vi "dialisis.vi"() -> ()   [LabVIEW 2014]
panel:
  out "T1":bool
  out "T2":bool
  out "TOXINS":dbl
  out "TOXINS":dbl(slide) scale=0.0..2000.0
  out "MILILITERS WATER":dbl
  out ".":bool
  out "1":bool
  out "Water to\nDialyzer":dbl(slide) scale=0.0..6000.0
  out "Boolean 4":bool
  out "Boolean 3":bool
  out "Boolean 2":bool
  out "Boolean":bool
  out "Manometer\nVenous Pressure\nmmHg":dbl(knob) scale=0.0..330.0
  out "Alarm V.P":bool
  in  "Venous\nPressure\nmmHg":dbl
  out "Alarm A.P":bool
  in  "Arterial\nPressure\nmmHg":dbl
  out "Manometer\nArterial Pressure\nmmHg":dbl(knob) scale=0.0..330.0
  out "TOXINES":dynamicdata(graph)
  out "MILILITERS\n VENOUS \nBLOOD":dbl
  out "MILILITERS\nARTERIAL\nBLOOD":dbl
  out "RETURN BLOOD WITH OUT TOXINS":dynamicdata(graph)
  out "FLOW BLOOD WITH TOXINS":dynamicdata(graph)
  in  "ON":bool
  out "Alarm TEMP":bool
  out "Thermometer":dbl(slide) scale=0.0..42.0
  out "Valve return blood":bool
  in  "BLOOD RETURN":dbl
  out "Air Valve":bool
  in  "Air Detector":bool
  out "MOTOR":bool
  in  "OFF":bool
  in  "INITIAL VALUE\nBLOD \nPATIENT":dbl
  out "Venous Blood":dbl(slide) scale=0.0..6000.0
  out "Arterial Blood":dbl(slide) scale=0.0..6000.0
  out "Valve":bool
  # "HEMODIALISIS MACHINE"
  # "HEMODIALYSIS\n MACHINE"
  # "Peristaltic motor"
  # "DIALYZER"
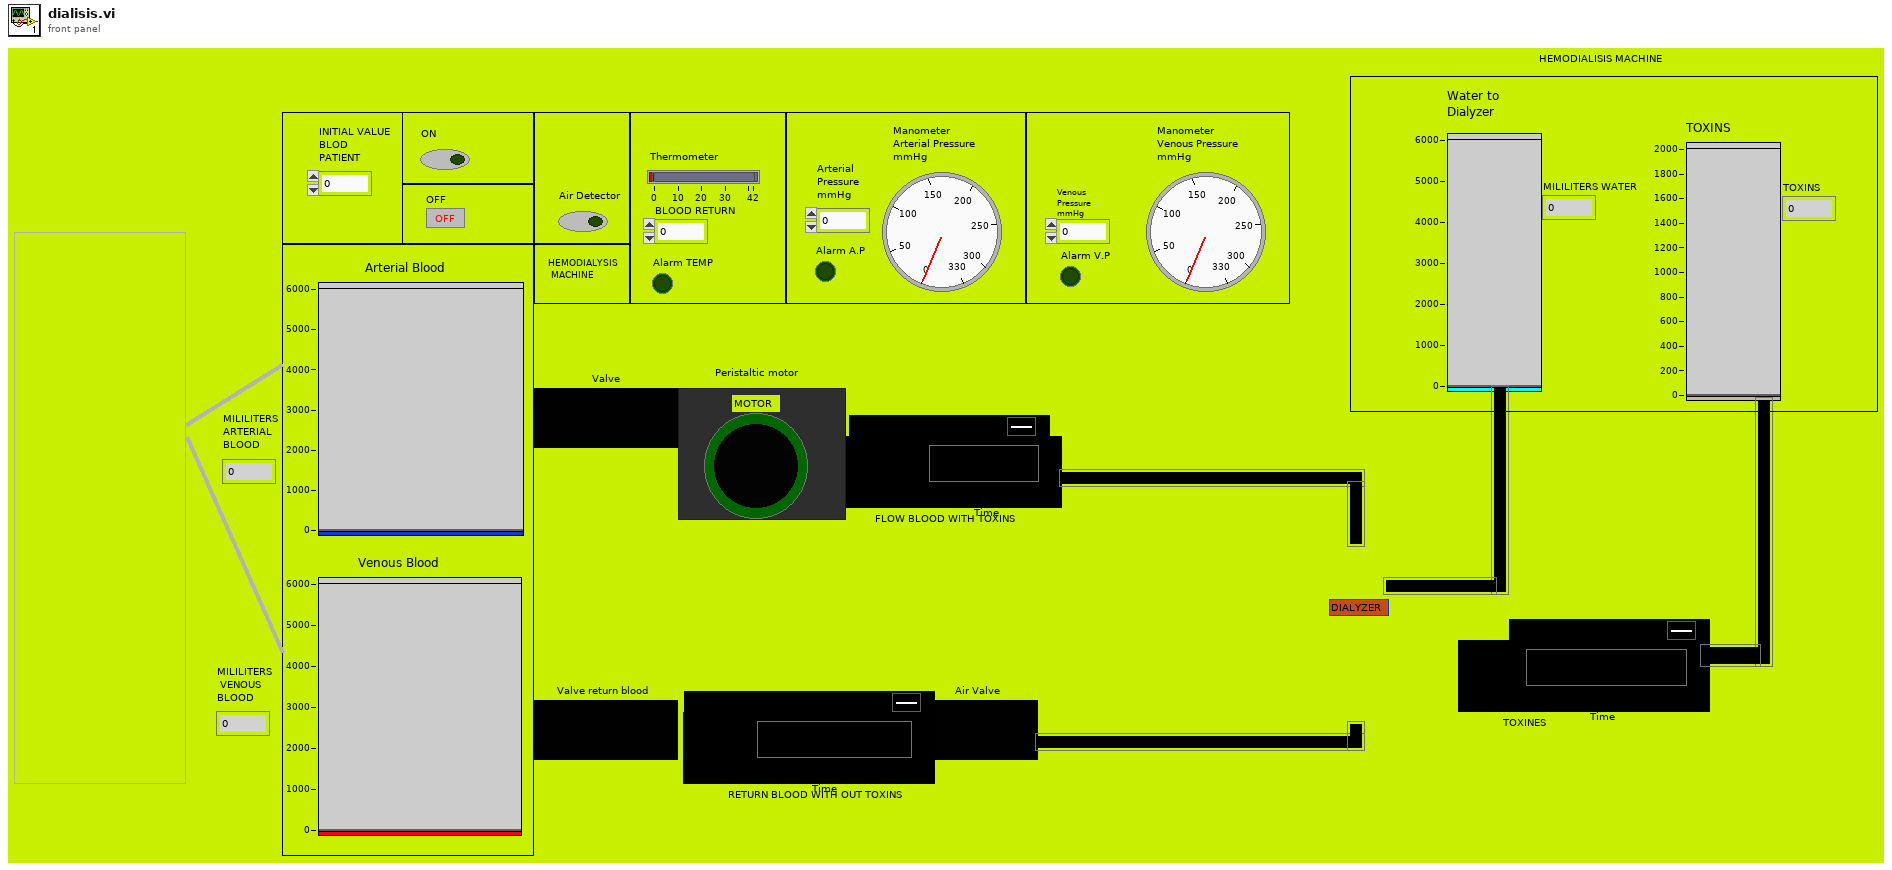
[diagram p1: front panel]
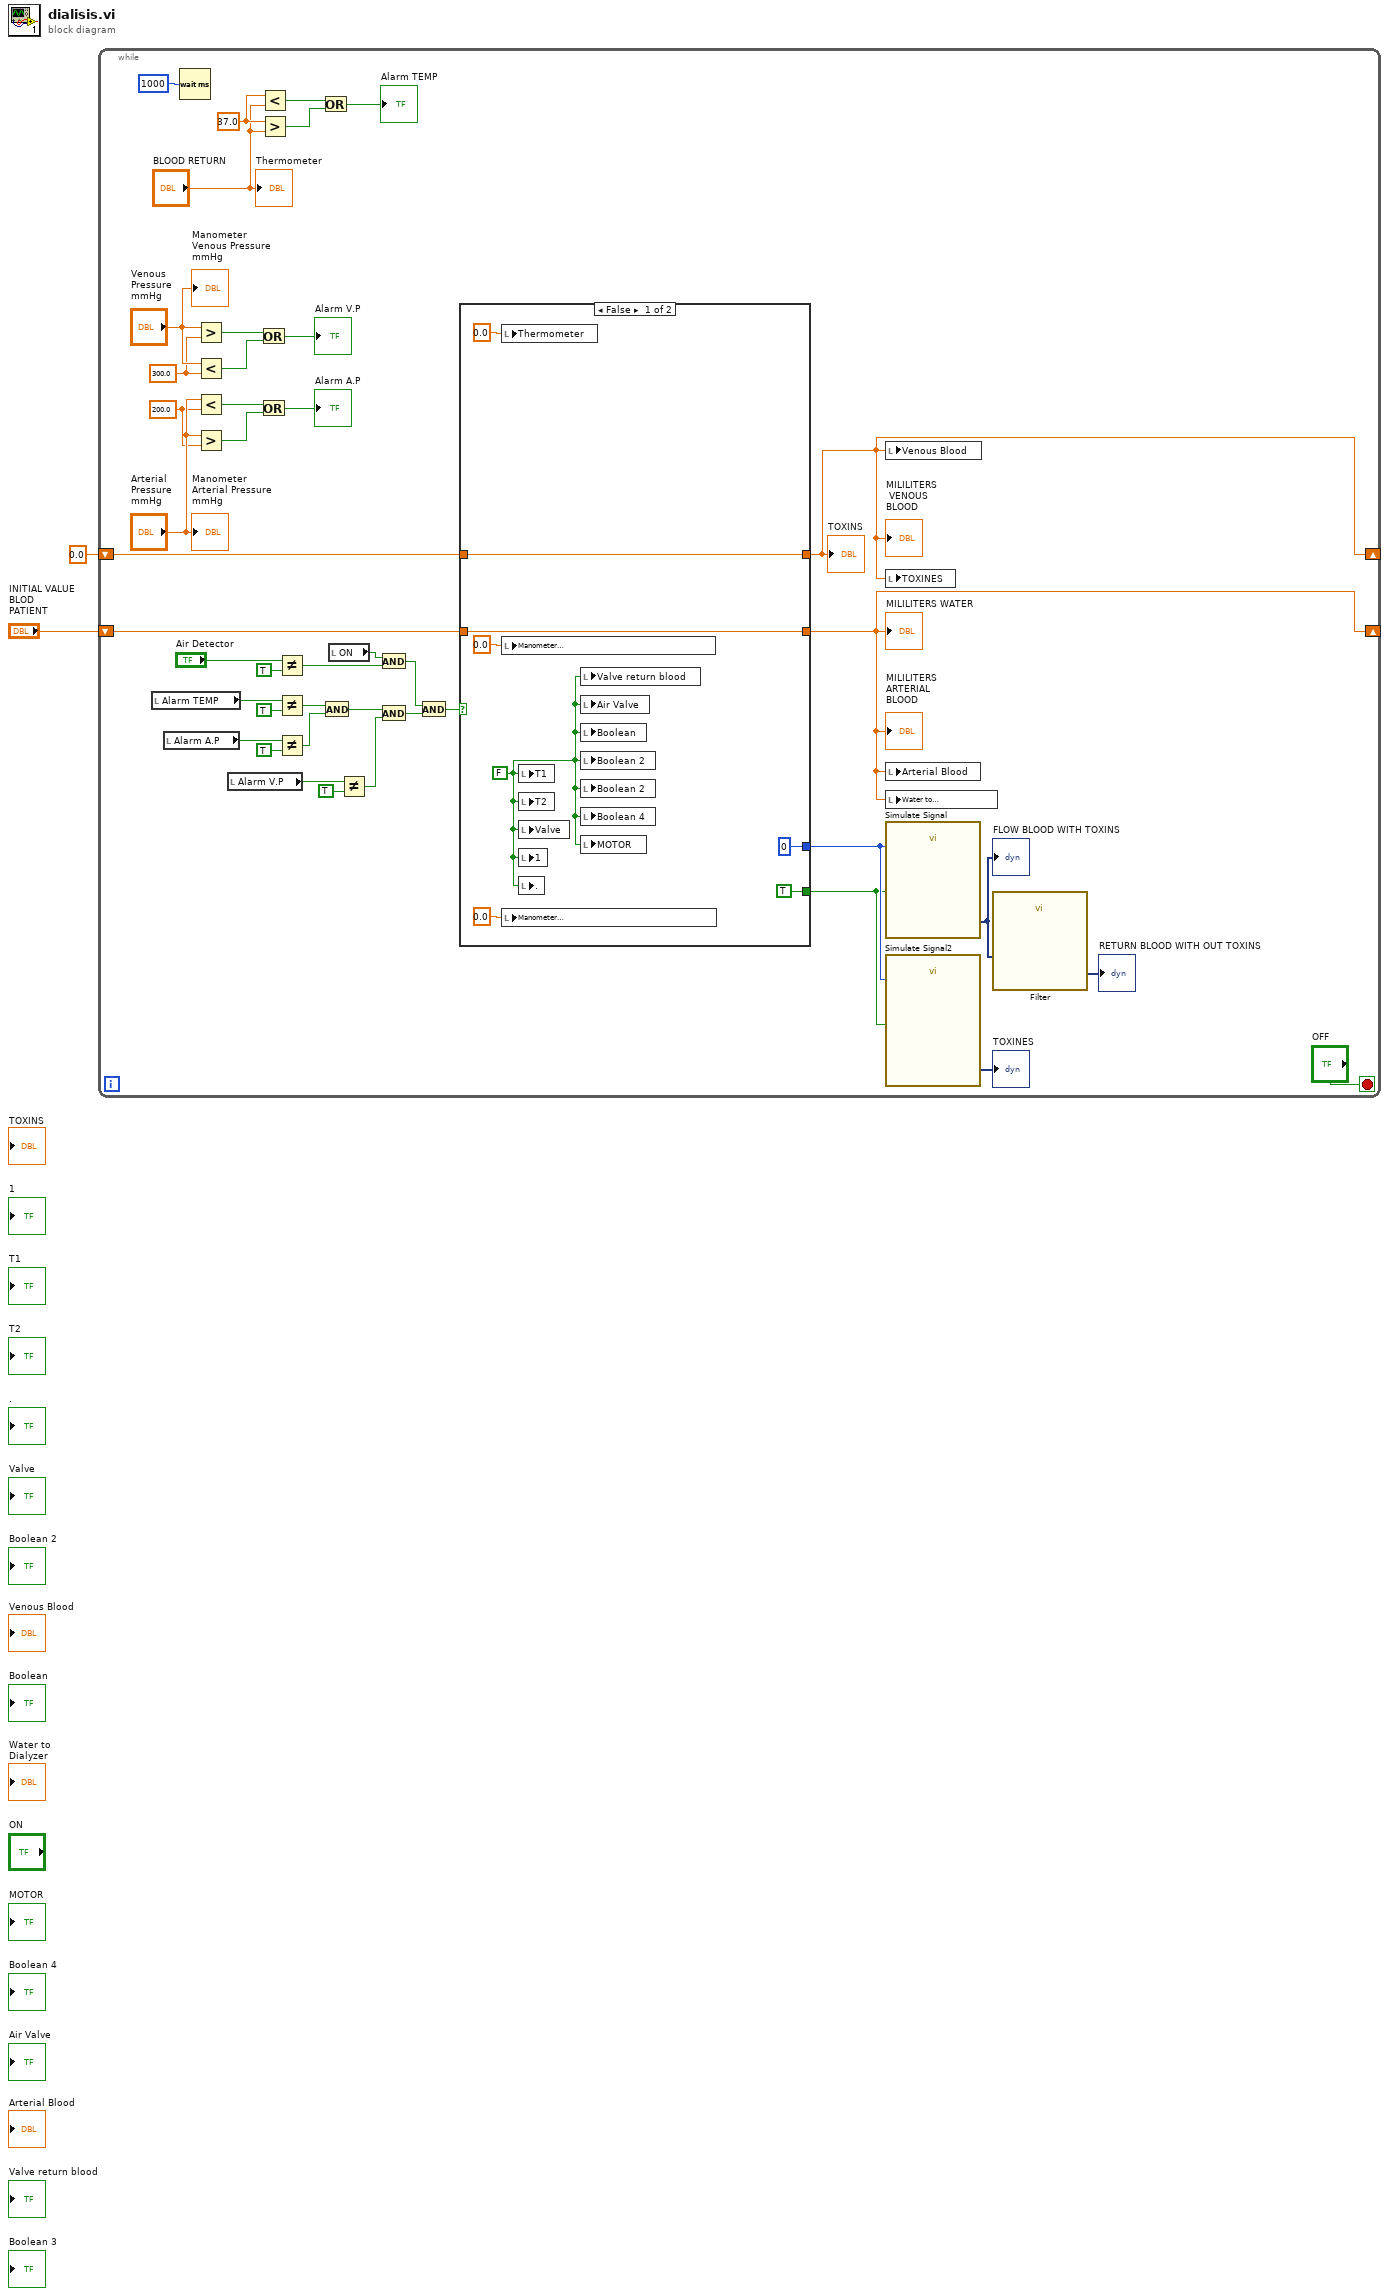
[diagram p0: block diagram]
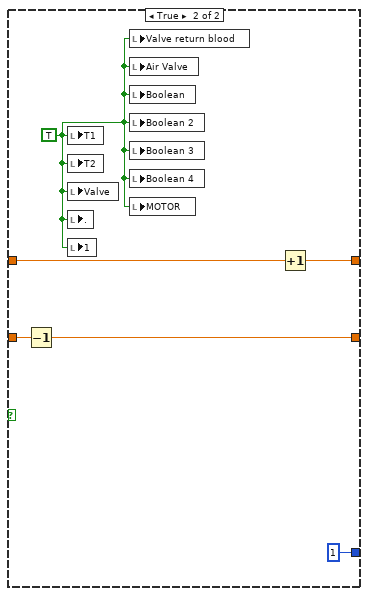
[diagram p2: hidden frame]
diagram:
  n1 = while {
    shift-right: [w5] -> _
    shift-left: "INITIAL VALUE\nBLOD \nPATIENT" -> [w37]
    shift-right: [w3] -> _
    shift-left: 0.0 -> [w4]
    stop <- "OFF" stop-if-true
    w20 = 300.0 ("y")
    w13 = 200.0 ("y")
    w32 = 37.0 ("x")
    n2 = local read "Alarm TEMP"() -> (w35:bool)
    n3 = local read "Alarm A.P"() -> (w25:bool)
    n4 = Wait (ms)(milliseconds to wait=u32 1000) -> ()  [unwired: 1 out]
    n5 = Greater?(x="Venous\nPressure\nmmHg", y=w20) -> (0:w12:bool)
    n6 = Less?(x="Venous\nPressure\nmmHg", y=w20) -> (x < y?=w11:bool)
    n7 = Less?(x="Arterial\nPressure\nmmHg", y=w13) -> (x < y?=w9:bool)
    n8 = Greater?(x="Arterial\nPressure\nmmHg", y=w13) -> (0:w8:bool)
    n9 = local read "Alarm V.P"() -> (w19:bool)
    n10 = Or(x=w12, y=w11) -> (x .or. y?=→"Alarm V.P":bool)
    n11 = Or(x=w9, y=w8) -> (x .or. y?=→"Alarm A.P":bool)
    n12 = Less?(x=w32, y="BLOOD RETURN") -> (x < y?=w33:bool)
    n13 = Greater?(x=w32, y="BLOOD RETURN") -> (0:w34:bool)
    n14 = Not Equal?(x="Air Detector", y=TRUE) -> (x != y?=w43:bool)
    n15 = Not Equal?(x=w35, y=TRUE) -> (x != y?=w23:bool)
    n16 = Not Equal?(x=w25, y=TRUE) -> (x != y?=w22:bool)
    n17 = Or(x=w33, y=w34) -> (x .or. y?=→"Alarm TEMP":bool)
    n18 = And(x=w23, y=w22) -> (x .and. y?=w17:bool)
    n19 = local read "ON"() -> (w44:bool)
    n20 = Not Equal?(x=w19, y=TRUE) -> (x != y?=w15:bool)
    n21 = And(x=w44, y=w43) -> (x .and. y?=w38:bool)
    n22 = And(x=w17, y=w15) -> (x .and. y?=w16:bool)
    n23 = And(x=w38, y=w16) -> (x .and. y?=w39:bool)
    n24 = case shown="False" w39 {
      tunnel: w4 -> [w53 w59]
      tunnel: w37 -> [w52 w58]
      tunnel: [w53 w57] -> w3
      tunnel: [w52 w56] -> w5
      tunnel: [0 1] -> w29
      tunnel: [TRUE ("Reset Signal") _] -> w28
      frame False {
        w46 = FALSE ("MOTOR")
        n25 = local write "Thermometer"(0.0 ("Thermometer")) -> ()
        n26 = local write "Manometer\nArterial Pressure\nmmHg"(0.0 ("Manometer\nArterial Pressure\nmmHg")) -> ()
        n27 = local write "Manometer\nVenous Pressure\nmmHg"(0.0 ("Manometer\nVenous Pressure\nmmHg")) -> ()
        n28 = local write "T1"(w46) -> ()
        n29 = local write "T2"(w46) -> ()
        n30 = local write "Valve"(w46) -> ()
        n31 = local write "1"(w46) -> ()
        n32 = local write "."(w46) -> ()
        n33 = local write "Valve return blood"(w46) -> ()
        n34 = local write "Air Valve"(w46) -> ()
        n35 = local write "Boolean"(w46) -> ()
        n36 = local write "Boolean 2"(w46) -> ()
        n37 = local write "Boolean 2"(w46) -> ()
        n38 = local write "Boolean 4"(w46) -> ()
        n39 = local write "MOTOR"(w46) -> ()
      }
      frame True {
        w54 = TRUE ("MOTOR")
        n40 = Decrement(x=w58) -> (x-1=w56:dbl)
        n41 = local write "T1"(w54) -> ()
        n42 = local write "T2"(w54) -> ()
        n43 = local write "Valve"(w54) -> ()
        n44 = local write "."(w54) -> ()
        n45 = local write "1"(w54) -> ()
        n46 = local write "Valve return blood"(w54) -> ()
        n47 = local write "Air Valve"(w54) -> ()
        n48 = local write "Boolean"(w54) -> ()
        n49 = local write "Boolean 2"(w54) -> ()
        n50 = local write "Boolean 3"(w54) -> ()
        n51 = local write "Boolean 4"(w54) -> ()
        n52 = local write "MOTOR"(w54) -> ()
        n53 = Increment(x=w59) -> (x+1=w57:dbl)
      }
    }
    "MILILITERS\n VENOUS \nBLOOD" <- w3
    "MILILITERS\nARTERIAL\nBLOOD" <- w5
    "MILILITERS WATER" <- w5
    "TOXINS" <- w3
    n54 = local write "Venous Blood"(w3) -> ()
    n55 = local write "TOXINES"(w3) -> ()
    n56 = local write "Arterial Blood"(w5) -> ()
    n57 = local write "Water to\nDialyzer"(w5) -> ()
    n58 = call "Simulate Signal"("Reset Signal"=w28, "Amplitude"=w29) -> ("Sine with Bernoulli Noise"=w26:dynamicdata)  [unwired: 12 in, 1 out]
    "FLOW BLOOD WITH TOXINS" <- w26
    n59 = call "Simulate Signal2"("Reset Signal"=w28, "Amplitude"=w29) -> ("Sine with Gaussian Noise"=→"TOXINES":dynamicdata)  [unwired: 12 in, 1 out]
    n60 = call "Filter"("Signal"=w26) -> ("Filtered Signal"=→"RETURN BLOOD WITH OUT TOXINS":dynamicdata)  [unwired: 9 in, 1 out]
    "Thermometer" <- "BLOOD RETURN"
    "Manometer\nArterial Pressure\nmmHg" <- "Arterial\nPressure\nmmHg"
    "Manometer\nVenous Pressure\nmmHg" <- "Venous\nPressure\nmmHg"
  }
